vi "Get Sphere S Aand Vol.vi"(11 "radius":dbl) -> (1 "function return":i32, 2 "vol":dbl, 3 "sa":dbl)   [LabVIEW 2018, in "Labview_to_DLL.lvlib"]
doc: "extern \"C\" __declspec(dllexport) int GetSphereSAandVol(double radius, double* sa, double* vol);"
uses:
  Labview_to_DLL.lvlib
  vs/Debug/Labview_to_DLL.dll
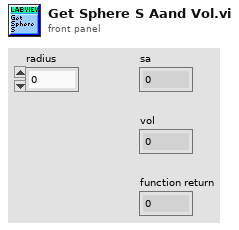
[diagram p1: front panel]
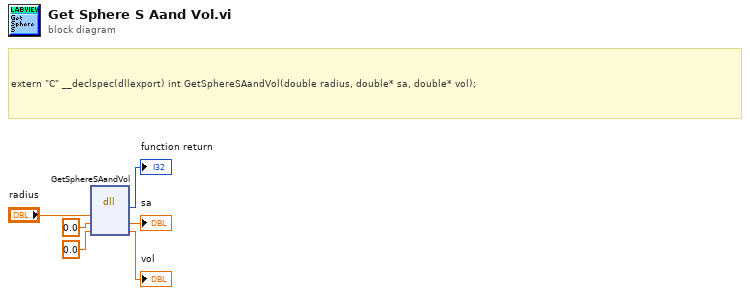
[diagram p0: block diagram]
diagram:
  # "extern \"C\" __declspec(dllexport) int GetSphereSAandVol(double radius, double* sa, double* vol);"
  n1 = dll-call lib="C:/Users/celit/Documents/GitHub/Labview_Python_DLL_Call/vs/Debug/Labview_to_DLL.*" fn="GetSphereSAandVol"("radius"="radius", "sa"=0.0, "vol"=0.0) -> (→"function return":i32, "sa"=→"sa":dbl, "vol"=→"vol":dbl)  [unwired: 4 in, 2 out]
